vi "TestTriggerModule.vi"() -> ()   [LabVIEW 2017]
uses:
  <vilib>/addons/Qbus/Qbus.lvclass
  <vilib>/addons/Qbus/controls/state.ctl
  <vilib>/addons/InsightCM/Devices/Shared/Common/Trigger/Trigger.lvlib
  <vilib>/addons/TimerProcess/TimerProcess.lvlib
  <vilib>/addons/WatchdogProcess/WatchdogProcess.lvlib
  <vilib>/addons/InsightCM/Devices/Shared/Common/TracePointDisplay/TracePointDisplay.lvlib
  <vilib>/addons/InsightCM/Devices/Shared/Common/ScanEngine/ScanEngine.lvlib
  <vilib>/addons/InsightCM/Utilities/GlobalConfiguration/GlobalConfiguration.lvlib
  <vilib>/addons/InsightCM/MessageBus/MessageLibrary/Device/controls/DeviceForceTriggerRoutedMessageBody.ctl
  <vilib>/addons/InsightCM/Devices/Shared/Common/Controller/Controller.lvlib
panel:
  in  "DataGroup":string
  in  "ForceTrigger":bool
  in  "Next":bool
  in  "Continous":bool
  out "ControllerLog":string
  out "error out":errorcluster
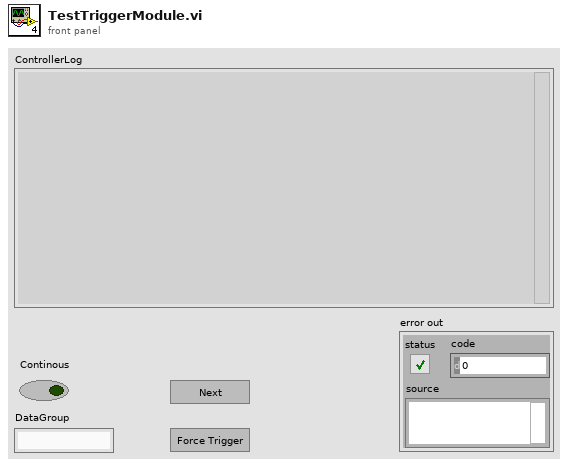
[diagram p1: front panel]
types:
  T1 = typedef "ScanEngine.lvlib/SimConfigRefs.ctl" = cluster{"Scan Engine Config":refnum<vi>}
  T2 = typedef "Qbus.lvclass/state.ctl" = enum16{"unconfigured", "configured"}
  T3 = typedef "DeviceForceTriggerRoutedMessageBody.ctl" = cluster{"DataGroup":string}
  T4 = typedef "ScanEngine.lvlib/Configuration.ctl" = cluster{"DynamicFPGAVIRef":refnum<k20>, "Device":string, "Groups":T5[]}
  T5 = typedef "ScanEngine.lvlib/Group.ctl" = cluster{"Group":string, "Channels":T6[]}
  T6 = typedef "ScanEngine.lvlib/Channel.ctl" = cluster{"Name":string, "Hardware Channel":string, "ChannelType":string, "TrendPoint Id":string, "Value":sgl, "Slope":dbl, "Offset":dbl, "IO variable":refnum<k21>, "datatype":T7, "Properties":T8[]}
  T7 = typedef "NI_Data Type.lvlib/Data Type.ctl" = enum8{"Invalid Type", "Void", "I8", "I16", "I32", "I64", "U8", "U16", "U32", "U64", "Single Float", "Double Float", "Extended Float", "Single Complex", "Double Complex", "Extended Complex", "Enum U8", "Enum U16", "Enum U32", "Enum U64", "Single Float With Unit", "Double Float With Unit", "Extended Float With Unit", "Single Complex with Unit", "Double Complex with Unit", "Extended Complex with Unit", "Boolean", "String", "Path", "Picture", "Tag", "Array", "Cluster", "Variant", "LV Variant", "Waveform", "Timestamp", "Digital Waveform", "Digital Data", "ExpressData", "Refnum", "External Data", "VI", "Poly VI", "LabVIEW Class Instance", "Fixed Point"}
  T8 = typedef "KeyValuePair.ctl" = cluster{"Key":string, "Value":string}
  T9 = typedef "Message.ctl" = cluster{"Header":T10, "Body":u8[]}
  T10 = typedef "MessageHeader.ctl" = cluster{"MessageName":string, "Timestamp":i64, "CorrelationId":string, "ContentType":string, "RoutingKey":string, "Properties":T8[]}
  T11 = typedef "PointValueMap.lvlib/PointMap.ctl" = refnum<data-value>
  T12 = typedef "AnalysisHelper.lvlib/PulsePositions.ctl" = cluster{"Name":string, "Pulse Position Data":dbl[], "Pulses Per Rev":i32}
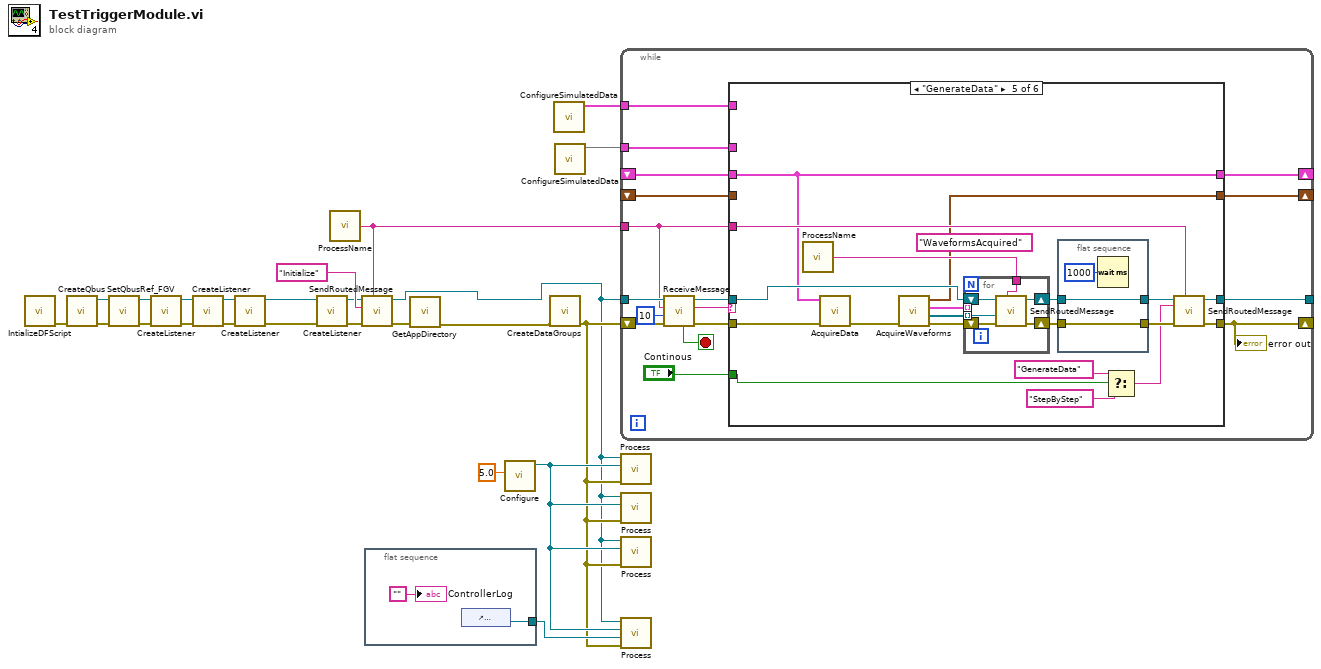
[diagram p0: block diagram]
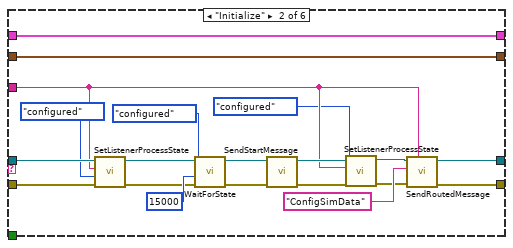
[diagram p3: hidden frame]
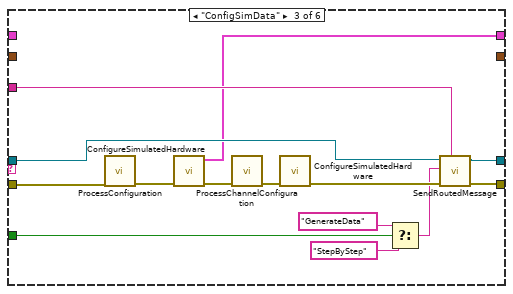
[diagram p4: hidden frame]
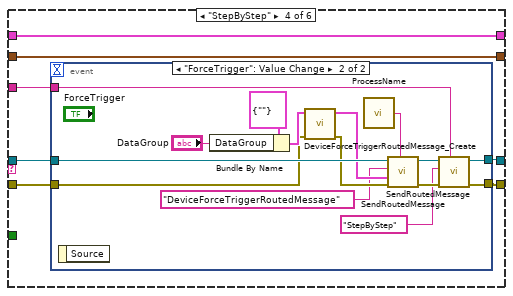
[diagram p5: hidden frame]
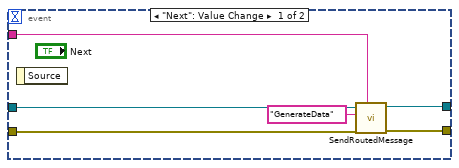
[diagram p6: hidden frame]
diagram:
  n1 = call <vilib>:"IntializeDFScript.vi"() -> ("error out"=w17:errorcluster)  [unwired: 11 in]
  n2 = call <vilib>:"CreateQbus.vi"("error in (no error)"=w17) -> ("error out"=w20:errorcluster, "Qbus"=w21:refnum<class "Qbus.lvclass">)  [unwired: 9 in]
  n3 = call <vilib>:"SetQbusRef_FGV.vi"("error in (no error)"=w20, "Qbus in"=w21) -> ("error out"=w22:errorcluster, "Qbus out"=w23:refnum<class "Qbus.lvclass">)  [unwired: 8 in]
  n4 = call <vilib>:"CreateListener.vi"("error in (no error)"=w22, "Qbus in"=w23) -> ("error out"=w12:errorcluster, "Qbus out"=w13:refnum<class "Qbus.lvclass">)  [unwired: 8 in]
  n5 = call <vilib>:"CreateListener.vi"("error in (no error)"=w12, "Qbus"=w13) -> ("error out"=w10:errorcluster, "Qbus out"=w11:refnum<class "Qbus.lvclass">)  [unwired: 8 in]
  n6 = call <vilib>:"CreateListener.vi"("error in (no error)"=w10, "Qbus in"=w11) -> ("error out"=w2:errorcluster, "Qbus out"=w1:refnum<class "Qbus.lvclass">)  [unwired: 8 in]
  n7 = call <vilib>:"CreateListener.vi"("error in (no error)"=w2, "qbus in"=w1) -> ("error out"=w8:errorcluster, "qbus out"=w9:refnum<class "Qbus.lvclass">)  [unwired: 8 in]
  n8 = call <vilib>:"ProcessName.vi"() -> ("ProcessName"=w19:string)  [unwired: 5 in]
  n9 = call <vilib>:"SendRoutedMessage.vi"("listener process"=w19, "error in (no error)"=w8, "message name"="Initialize" ("ProcessName"), "Qbus in"=w9) -> ("error in (no error)"=w7:errorcluster, "Qbus out"=w3:refnum<class "Qbus.lvclass">)  [unwired: 6 in]
  n10 = flat-sequence {
    tunnel: [w26] -> w16
    frame #0 {
      n11 = control-ref of="ControllerLog"() -> (w26:refnum<vi>)
      "ControllerLog" <- ""
    }
  }
  n12 = call <vilib>:"GetAppDirectory.vi"("error in (no error)"=w7) -> ("error out"=w4:errorcluster)  [unwired: 9 in, 1 out]
  n13 = call <vilib>:"Configure.vi"("hw timeout (sec)"=5.0) -> ("Pound"=w15:refnum<class "Pound.lvclass">)  [unwired: 8 in, 2 out]
  n14 = call <vilib>:"CreateDataGroups.vi"("error in (no error)"=w4) -> ("error out"=w14:errorcluster)  [unwired: 10 in]
  n15 = call <vilib>:"ConfigureSimulatedData.vi"() -> ("Sim Config Refs"=w6:T1)  [unwired: 11 in]
  n16 = call <vilib>:"ConfigureSimulatedData.vi"() -> (3:w5)  [unwired: 11 in]
  n17 = while {
    shift-right: [w39] -> _
    shift-left: w14 -> [w43]
    tunnel: [w37] -> _
    tunnel: w3 -> [w36]
    tunnel: w19 -> [w34]
    shift-right: [w32] -> _
    shift-left: _ -> [w31]
    shift-right: [w33] -> _
    shift-left: _ -> [w30]
    tunnel: w6 -> [w29]
    tunnel: w5 -> [w28]
    stop <- w35 stop-if-true
    n18 = call <vilib>:"ReceiveMessage.vi"("error in (no error)"=w43, "timeout (0)"=10, "process name"=w34, "Qbus in"=w36) -> ("error in (no error)"=w41:errorcluster, "message name"=w38:string, "Qbus out"=w40:refnum<class "Qbus.lvclass">, "exit"=w35:bool)  [unwired: 2 in, 2 out]
    n19 = case shown="\"GenerateData\"" w38 {
      tunnel: w41 -> [w46 w65 w78 w85 w121 w141]
      tunnel: w40 -> [w47 w64 w73 w86 w120 w142]
      tunnel: [w46 w49 w80 w83 w126 w141] -> w39
      tunnel: [w47 w48 w81 w84 w127 w142] -> w37
      tunnel: w34 -> [_ w55 w79 w82 w123 _]
      tunnel: w29 -> [_ _ _ _ _ _]
      tunnel: w28 -> [_ _ _ _ _ _]
      tunnel: [w44 w53 _ w88 w116 w139] -> w33
      tunnel: [w45 w54 w72 w87 w117 w140] -> w32
      tunnel: w31 -> [w45 w54 _ w87 w117 w140]
      tunnel: w30 -> [w44 w53 _ w88 _ w139]
      tunnel: "Continous" -> [_ _ w68 _ w110 _]
      frame "False", Default {
      }
      frame "Initialize" {
        n20 = call <vilib>:"SetListenerProcessState.vi"("error in (no error)"=w65, "state"=state."configured", "process name"=w55, "Qbus in"=w64) -> ("error in (no error)"=w62:errorcluster, "Qbus out"=w63:refnum<class "Qbus.lvclass">)  [unwired: 6 in]
        n21 = call <vilib>:"WaitForState.vi"("error in (no error)"=w62, "timeout (-1)"=15000, "state"=state."configured", "Qbus in"=w63) -> ("error in (no error)"=w60:errorcluster, "Qbus out"=w61:refnum<class "Qbus.lvclass">)  [unwired: 4 in, 2 out]
        n22 = call <vilib>:"SendStartMessage.vi"("error in (no error)"=w60, "Qbus in"=w61) -> ("error in (no error)"=w59:errorcluster, "Qbus out"=w58:refnum<class "Qbus.lvclass">)  [unwired: 8 in]
        n23 = call <vilib>:"SetListenerProcessState.vi"("error in (no error)"=w59, "state"=state."configured", "process name"=w55, "Qbus in"=w58) -> ("error in (no error)"=w57:errorcluster, "Qbus out"=w56:refnum<class "Qbus.lvclass">)  [unwired: 6 in]
        n24 = call <vilib>:"SendRoutedMessage.vi"("listener process"=w55, "error in (no error)"=w57, "message name"="ConfigSimData" ("MsgName"), "Qbus in"=w56) -> ("error in (no error)"=w49:errorcluster, "Qbus out"=w48:refnum<class "Qbus.lvclass">)  [unwired: 6 in]
      }
      frame "ConfigSimData" {
        n25 = call <vilib>:"ProcessConfiguration.vi"("error in (no error)"=w78) -> ("error out"=w75:errorcluster)  [unwired: 7 in, 3 out]
        n26 = call <vilib>:"ConfigureSimulatedHardware.vi"("error in (no error)"=w75) -> ("error out"=w76:errorcluster, "Scan Engine Config Out"=w72:T4)  [unwired: 9 in]
        n27 = call <vilib>:"ProcessChannelConfiguration.vi"("error in (no error)"=w76) -> ("error out"=w77:errorcluster)  [unwired: 7 in, 3 out]
        n28 = call <vilib>:"ConfigureSimulatedHardware.vi"("error in (no error)"=w77) -> ("error out"=w74:errorcluster)  [unwired: 9 in, 1 out]
        n29 = Select(t="GenerateData" ("MsgName"), s=w68, f="StepByStep" ("MsgName")) -> (s? t:f=w70:string)
        n30 = call <vilib>:"SendRoutedMessage.vi"("listener process"=w79, "error in (no error)"=w74, "message name"=w70, "Qbus in"=w73) -> ("error in (no error)"=w80:errorcluster, "Qbus out"=w81:refnum<class "Qbus.lvclass">)  [unwired: 6 in]
      }
      frame "StepByStep" {
        n31 = event shown="[1] \"ForceTrigger\": Value Change" {
          selector: _ -> [_ _]
          dyn-events: _ -> [_ _]
          timeout: _ -> [_ _]
          tunnel: w86 -> [w94 w109]
          tunnel: w85 -> [w93 w105]
          tunnel: [w92 w98] -> w84
          tunnel: [w91 w97] -> w83
          tunnel: w82 -> [w90 w96]
          event "Next": Value Change {
            n32 = event-data() -> ()  [unwired: 1 in, 1 out]
            n33 = call <vilib>:"SendRoutedMessage.vi"("listener process"=w90, "error in (no error)"=w93, "message name"="GenerateData" ("MsgName"), "Qbus in"=w94) -> ("error in (no error)"=w91:errorcluster, "Qbus out"=w92:refnum<class "Qbus.lvclass">)  [unwired: 6 in]
          }
          event "ForceTrigger": Value Change {
            n34 = event-data() -> ()  [unwired: 1 in, 1 out]
            n35 = Bundle By Name(cluster=T3 {"DataGroup"=""} ("DeviceForceTriggerRoutedMessage"), "DataGroup"="DataGroup") -> (w107:T3)
            n36 = call <vilib>:"DeviceForceTriggerRoutedMessage_Create.vi"("error in (no error)"=w105, "DeviceForceTriggerRoutedMessage"=w107) -> ("error out"=w104:errorcluster, "Message"=w103:T9)  [unwired: 8 in]
            n37 = call <vilib>:"ProcessName.vi"() -> ("process name"=w101:string)  [unwired: 5 in]
            n38 = call <vilib>:"SendRoutedMessage.vi"("listener process"=w101, "error in (no error)"=w104, "message value"=w103, "message name"="DeviceForceTriggerRoutedMessage" ("MsgName"), "Qbus in"=w109) -> ("error in (no error)"=w100:errorcluster, "Qbus out"=w99:refnum<class "Qbus.lvclass">)  [unwired: 5 in]
            n39 = call <vilib>:"SendRoutedMessage.vi"("listener process"=w96, "error in (no error)"=w100, "message name"="StepByStep" ("MsgName"), "Qbus in"=w99) -> ("error in (no error)"=w97:errorcluster, "Qbus out"=w98:refnum<class "Qbus.lvclass">)  [unwired: 6 in]
          }
        }
      }
      frame "GenerateData" {
        (unwired) "WaveformsAcquired" ("MsgName")
        n40 = call <vilib>:"ProcessName.vi"() -> ("ProcessName"=w122:string)  [unwired: 5 in]
        n41 = call <vilib>:"AcquireData.vi"("error in (no error)"=w121, "config in"=w117) -> ("error out"=w119:errorcluster)  [unwired: 8 in, 1 out]
        n42 = call <vilib>:"AcquireWaveforms.vi"("error in (no error)"=w119) -> ("error out"=w118:errorcluster, "Data Flow Maps out"=w115:T11[], "Pulse Positions Array"=w114:T12[], "Waveforms"=w116:waveform(sgl)[])  [unwired: 7 in]
        n43 = for {
          tunnel: w122 -> [w133]
          tunnel: w115 -> [w130] mode=indexing
          tunnel: w114 -> [_] mode=indexing
          shift-right: [w135] -> w125
          shift-left: w120 -> [w132]
          shift-right: [w134] -> w124
          shift-left: w118 -> [w131]
          n44 = call <vilib>:"SendRoutedMessage.vi"("listener process"=w133, "error in (no error)"=w131, "message value"=w130, "Qbus in"=w132) -> ("error in (no error)"=w134:errorcluster, "Qbus out"=w135:refnum<class "Qbus.lvclass">)  [unwired: 6 in]
        }
        n45 = flat-sequence {
          tunnel: w125 -> [w138]
          tunnel: w124 -> [w137]
          tunnel: [w138] -> w128
          tunnel: [w137] -> w129
          frame #0 {
            n46 = Wait (ms)(milliseconds to wait=u32 1000) -> ()  [unwired: 1 out]
          }
        }
        n47 = Select(t="GenerateData" ("MsgName"), s=w110, f="StepByStep" ("MsgName")) -> (s? t:f=w111:string)
        n48 = call <vilib>:"SendRoutedMessage.vi"("listener process"=w123, "error in (no error)"=w129, "message name"=w111, "Qbus in"=w128) -> ("error in (no error)"=w126:errorcluster, "Qbus out"=w127:refnum<class "Qbus.lvclass">)  [unwired: 6 in]
      }
      frame "ProcessError" {
      }
    }
    "error out" <- w39
  }
  n49 = call <vilib>:"Process.vi"("error in (no error)"=w14, "Pound in"=w15, "Qbus in"=w3) -> ()  [unwired: 8 in, 1 out]
  n50 = call <vilib>:"Process.vi"("error in (no error)"=w14, "Pound in"=w15, "Qbus in"=w3) -> ()  [unwired: 8 in, 1 out]
  n51 = call <vilib>:"Process.vi"("error in (no error)"=w14, "pound in"=w15, "qbus in"=w3) -> ()  [unwired: 8 in, 1 out]
  n52 = call <vilib>:"Process.vi"("error in (no error)"=w14, "string refnum"=w16, "Pound in"=w15, "Qbus in"=w3) -> ()  [unwired: 7 in, 1 out]
